vi "SetImage.vi"(1 "yoffset":i32, 2 "xoffset":i32, 3 "Image":T1, 4 "tracker":u64) -> (0 "tracker":u64)   [LabVIEW 2011]
uses:
  <vilib>/vision/Image Controls.llb/IMAQ Image.ctl
  TrackerDLL.vi
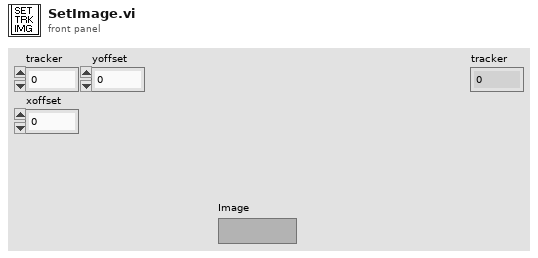
[diagram p1: front panel]
types:
  T1 = typedef "IMAQ Image.ctl" = refnum<image>
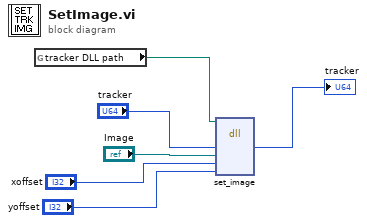
[diagram p0: block diagram]
diagram:
  n1 = global read "TrackerDLL.vi" "tracker DLL path"() -> (w1:path)
  n2 = dll-call lib="D:/jcnossen1/cudaqi-tracker/cudatrack-labview/cputrack.dll" fn="set_image"(path in=w1, "tracker"="tracker", "image"="Image", "xoffset"="xoffset", "yoffset"="yoffset") -> ("tracker"=→"tracker":u64)  [unwired: 6 in, 2 out]
